vi "SubVI server balance.vi"(10 "before match":string, 11 "appended path":path) -> (3 "String":string)   [LabVIEW 2020]
uses:
  <vilib>/Utility/file.llb/Read Delimited Spreadsheet (string).vi
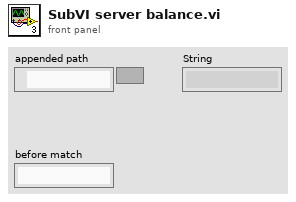
[diagram p1: front panel]
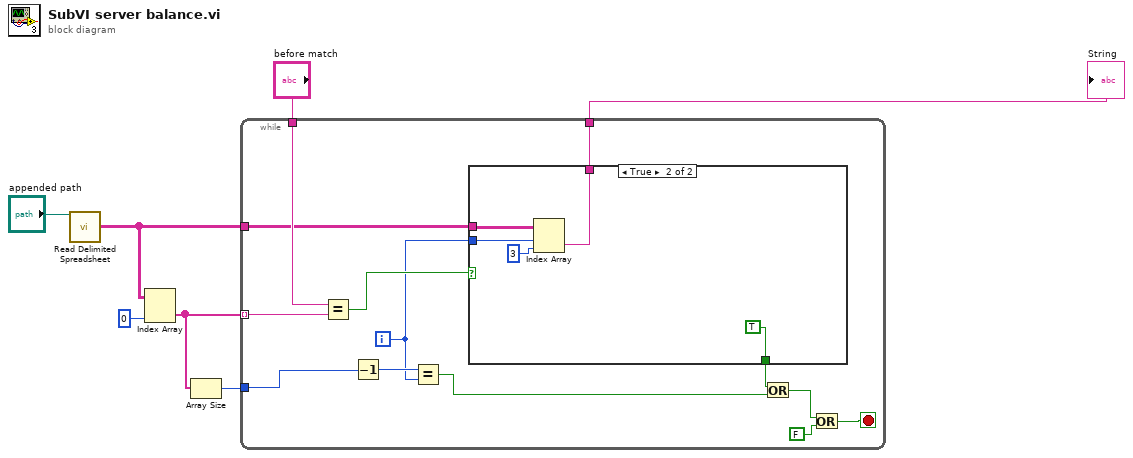
[diagram p0: block diagram]
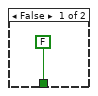
[diagram p2: hidden frame]
diagram:
  n1 = call-poly <vilib>:"Read Delimited Spreadsheet.vi"("file path (dialog if empty)"="appended path") -> ("all rows"=w3:string[][])  [unwired: 9 in, 5 out]
  n2 = Index Array "Index Array"(array=w3, index (col)=0 ("disabled index (col)")) -> (element=w4:string[])  [unwired: 1 in]
  n3 = Array Size(array=w4) -> (size(s)=w6:i32)
  n4 = while {
    tunnel: w3 -> [w14]
    tunnel: w4 -> [w17] mode=indexing
    tunnel: "before match" -> [w16]
    tunnel: w6 -> [w13]
    tunnel: [w11] -> w7
    i -> [w12]
    stop <- w18 stop-if-true
    n5 = Equal?(x=w16, y=w17) -> (x = y?=w15:bool)
    n6 = Decrement(x=w13) -> (x-1=w19:i32)
    n7 = Equal?(x=w19, y=w12) -> (x = y?=w9:bool)
    n8 = case shown="True" w15 {
      tunnel: w14 -> [_ w25]
      tunnel: w12 -> [_ w24]
      tunnel: [_ w23] -> w11
      tunnel: [FALSE TRUE] -> w8
      frame False {
      }
      frame True {
        n9 = Index Array "Index Array"(array=w25, index (row)=w24, index (col)=3 ("disabled index (col)")) -> (element=w23:string)
      }
    }
    n10 = Or(x=w8, y=w9) -> (x .or. y?=w10:bool)
    n11 = Or(x=w10, y=FALSE) -> (x .or. y?=w18:bool)
  }
  "String" <- w7
